vi "Get Diagram By ID.vi"(8 "error in (no error)":errorcluster, 10 "ID":i32, 11 "Data Cluster in":T1) -> (0 "error out":errorcluster, 2 "Diagram":refnum<vi>, 3 "Data Cluster out":T1)   [LabVIEW 2025, in "Scripting Server.lvlib"]
uses:
  Scripting Server.lvlib
  Module Data--cluster.ctl
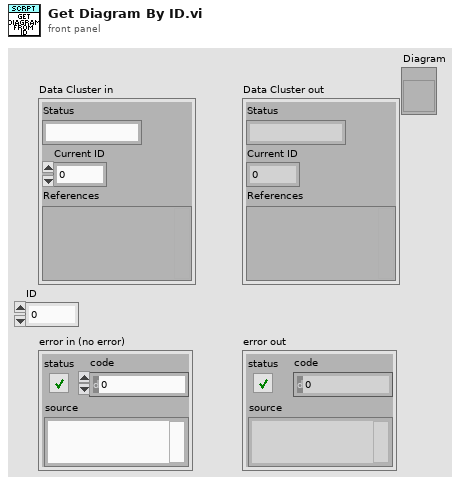
[diagram p1: front panel]
types:
  T1 = typedef "Scripting Server.lvlib/Module Data--cluster.ctl" = cluster{"Status":string, "Current ID":i32, "References":variant}
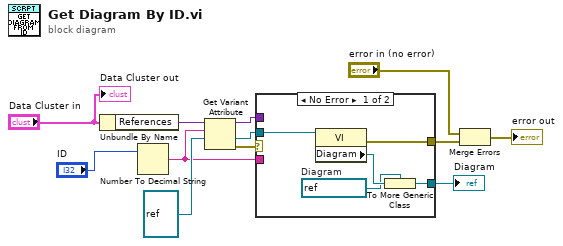
[diagram p0: block diagram]
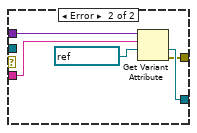
[diagram p2: hidden frame]
diagram:
  n1 = Unbundle By Name("Data Cluster in") -> ("References"=w12:variant)
  n2 = Number To Decimal String(number="ID") -> (decimal integer string=w5:string)  [unwired: 1 in]
  n3 = Get Variant Attribute(Variant=w12, name=w5, default value (empty Variant)=refnum<vi> refnum ("vi reference")) -> (duplicate Variant=w6:variant, value=w8:refnum<vi>, error out=w7:errorcluster)  [unwired: 1 in, 1 out]
  n4 = case shown="No Error" w7 {
    tunnel: w8 -> [w17 _]
    tunnel: [w15 w19] -> w1
    tunnel: w6 -> [_ w22]
    tunnel: w5 -> [_ w21]
    tunnel: [w13 w18] -> w2
    frame No Error {
      w14 = refnum<vi> refnum  # Diagram
      n5 = property class="VI"(reference=w17) -> (error out=w13:errorcluster, "Diagram"=w16:refnum<vi>)  [unwired: 1 in, 1 out]
      n6 = To More Generic Class(target class=w14, reference=w16) -> (generic class reference=w15:refnum<vi>)
    }
    frame Error {
      n7 = Get Variant Attribute(Variant=w22, name=w21, default value (empty Variant)=refnum<vi> refnum ("Diagram")) -> (value=w19:refnum<vi>, error out=w18:errorcluster)  [unwired: 1 in, 2 out]
    }
  }
  "Diagram" <- w1
  n8 = Merge Errors("error in (no error)", w2) -> (→"error out":errorcluster)
  "Data Cluster out" <- "Data Cluster in"
